vi "testAppendErrorInformation_Error_withState.vi"(8 "error in (no error)":errorcluster, 11 "testStateMachineUtilities in":refnum<class "testStateMachineUtilities.lvclass">) -> (0 "error out":errorcluster, 3 "testStateMachineUtilities out":refnum<class "testStateMachineUtilities.lvclass">)   [LabVIEW 2013, in "testStateMachineUtilities.lvclass"]
uses:
  testStateMachineUtilities.lvclass
  source/State Machine Support API/Parse State Queue_2024.vi
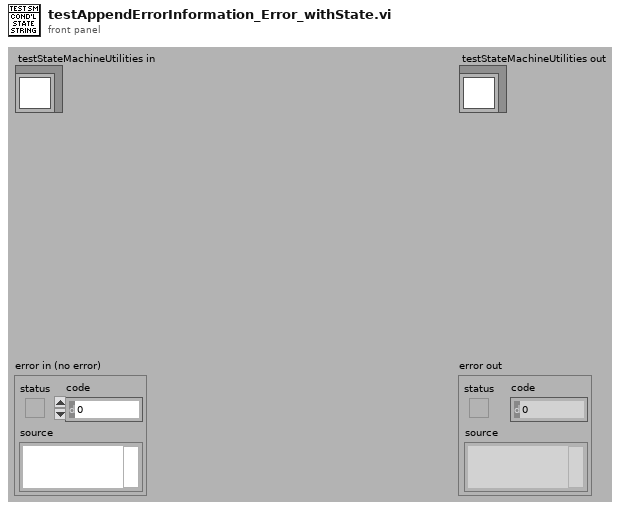
[diagram p1: front panel]
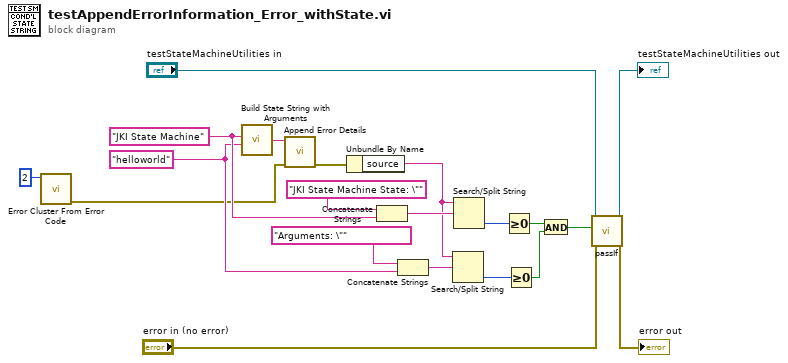
[diagram p0: block diagram]
diagram:
  w14 = "JKI State Machine" ("Previous State and Argument(s)")
  w12 = "helloworld" ("Previous State and Argument(s)")
  n1 = call <vilib>:"Error Cluster From Error Code.vi"("error code (0)"=2) -> ("error out"=w4:errorcluster)  [unwired: 8 in]
  n2 = call "Build State String with Arguments.vi"("Arguments (\"\")"=w12, "State"=w14) -> ("State with Arguments"=w16:string)  [unwired: 4 in]
  n3 = call "Append Error Details.vi"("error in (no error)"=w4, "Previous State and Argument(s)"=w16) -> ("error out"=w3:errorcluster)  [unwired: 9 in]
  n4 = Unbundle By Name(w3) -> ("source"=w2:string)
  n5 = Concatenate Strings("JKI State Machine State: \"" ("search string/char (-)"), w14) -> (w9:string)
  n6 = Concatenate Strings("Arguments: \"" ("search string/char (-)"), w12) -> (w8:string)
  n7 = Search/Split String(string=w2, search string/char (-)=w8) -> (offset of match=w10:i32)  [unwired: 1 in, 2 out]
  n8 = Search/Split String(string=w2, search string/char (-)=w9) -> (offset of match=w13:i32)  [unwired: 1 in, 2 out]
  n9 = Greater Or Equal To 0?(x=w13) -> (x >= 0?=w7:bool)
  n10 = Greater Or Equal To 0?(x=w10) -> (x >= 0?=w6:bool)
  n11 = And(x=w7, y=w6) -> (x .and. y?=w1:bool)
  n12 = call-dynamic "passIf.vi"("error in (no error)"="error in (no error)", "pass"=w1, "TestCase in"="testStateMachineUtilities in") -> ("error out"=→"error out":errorcluster, "TestCase out"=→"testStateMachineUtilities out":refnum<class "testStateMachineUtilities.lvclass">)  [unwired: 7 in]
